vi "Decimate Graph Data.vi"   [LabVIEW 2013, in "Workspace MultiY Graph.lvlib"]
uses:
  Workspace MultiY Graph.lvlib
  <vilib>/Analysis/2dsp.llb/Decimate (continuous, DBL).vi
  <vilib>/Analysis/NI_AALPro.lvlib
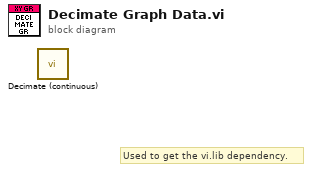
[diagram p0: block diagram]
diagram:
  # "Used to get the vi.lib dependency."
  n1 = call-poly <vilib>:"Decimate (continuous).vi"() -> ()  [unwired: 10 in, 2 out]
